vi "Dispose__slk_tc.vi"(0 "tree control in":refnum<class "TreeControl.lvclass">, 11 "error in (no error)":errorcluster) -> (15 "error out":errorcluster)   [LabVIEW 2020, in "TreeControl.lvclass"]
doc: "Disposes TREE CONTROL object."
uses:
  Library/TreeControl.lvclass
  Library/TreeControl.lvclass/TreeControl.ctl
panel:
  out "tree control out":refnum<class "TreeControl.lvclass">
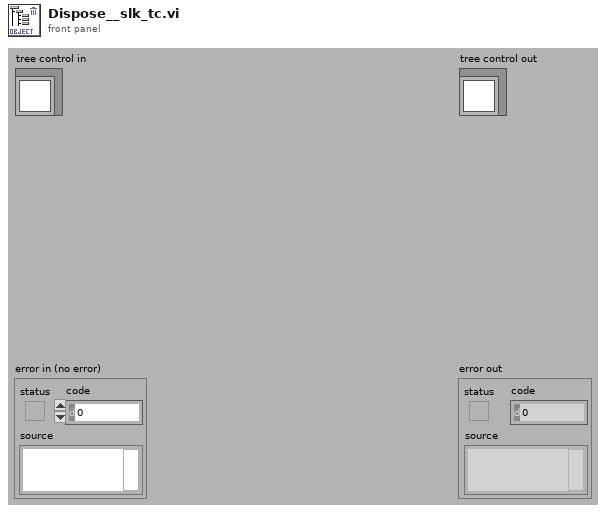
[diagram p1: front panel]
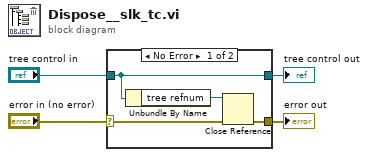
[diagram p0: block diagram]
diagram:
  n1 = case shown="No Error" "error in (no error)" {
    selector: "error in (no error)" -> [w8 w10]
    tunnel: [w6 w10] -> w3
    tunnel: [w7 w9] -> w1
    tunnel: "tree control in" -> [w7 w9]
    frame No Error {
      n2 = Unbundle By Name(w7) -> ("tree refnum"=w5:refnum<vi>)
      n3 = Close Reference(reference=w5, error in (no error)=w8) -> (error out=w6:errorcluster)
    }
    frame Error {
    }
  }
  "error out" <- w3
  "tree control out" <- w1
